vi "AC concatentated string command.vi"(11 "MathCAD results":T1) -> (3 "AC concatenated string":string)   [LabVIEW 2015]
uses:
  Variable cluster.ctl
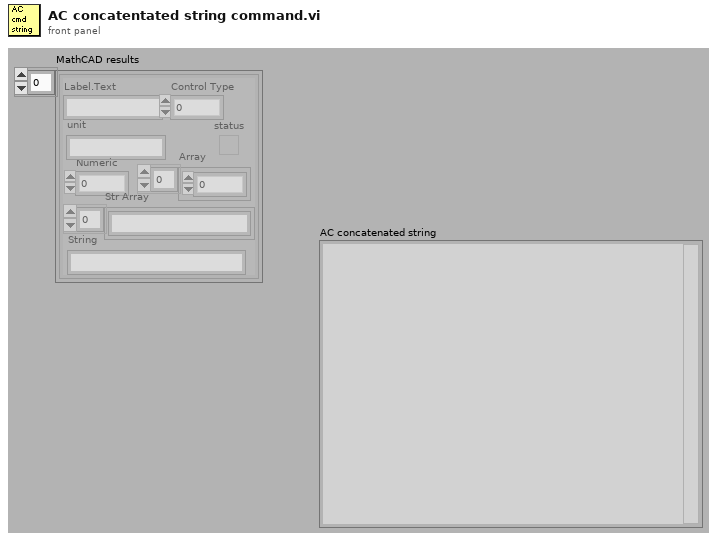
[diagram p1: front panel]
types:
  T1 = typedef "Variable cluster.ctl" = cluster{"Label.Text":string, "Control Type":u32, "Numeric":dbl, "Array":dbl[], "status":bool, "Str Array":string[], "String":string, "unit":string}[]
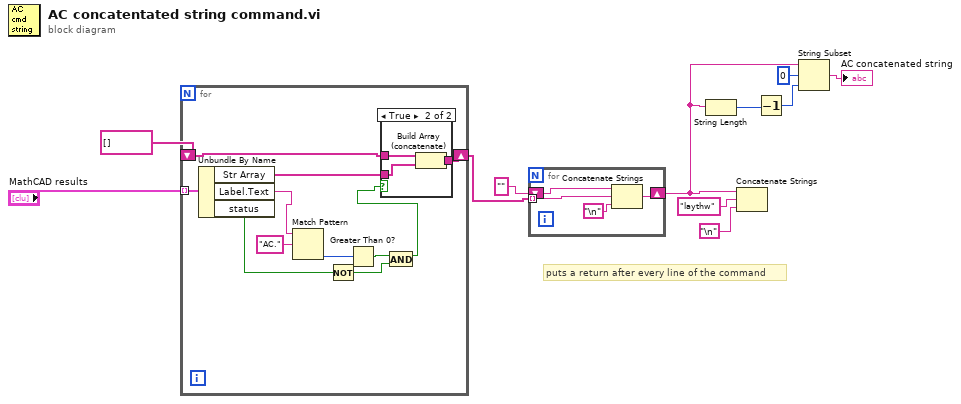
[diagram p0: block diagram]
diagram:
  # "puts a return after every line of the command"
  n1 = for {
    tunnel: "MathCAD results" -> [w22] mode=indexing
    shift-right: [w18] -> w8
    shift-left: string[] [] -> [w16]
    n2 = Unbundle By Name(w22) -> ("Str Array"=w13:string[], "Label.Text"=w21:string, "status"=w15:bool)
    n3 = Match Pattern(string=w21, regular expression="AC.") -> (offset past match=w19:i32)  [unwired: 1 in, 3 out]
    n4 = Not(x=w15) -> (.not. x?=w14:bool)
    n5 = Greater Than 0?(x=w19) -> (x > 0?=w17:bool)
    n6 = And(x=w17, y=w14) -> (x .and. y?=w12:bool)
    n7 = case shown="True" w12 {
      tunnel: [w23 w26] -> w18
      tunnel: w16 -> [w23 w25]
      tunnel: w13 -> [_ w24]
      frame False {
      }
      frame True {
        n8 = Build Array (concatenate)(w25, w24) -> (w26:string[])
      }
    }
  }
  n9 = for {
    tunnel: w8 -> [w30] mode=indexing
    shift-right: [w28] -> w2
    shift-left: "" -> [w29]
    n10 = Concatenate Strings(w29, w30, "\n") -> (w28:string)
  }
  n11 = String Length(string=w2) -> (length=w4:i32)
  n12 = Concatenate Strings(w2, "laythw", "\n") -> ()  [unwired: 1 out]
  n13 = Decrement(x=w4) -> (x-1=w3:i32)
  n14 = String Subset(string=w2, offset (0)=0, length (rest)=w3) -> (substring=→"AC concatenated string":string)
